vi "SwerveDriveLogic.vi"(8 "Z":dbl, 9 "Speeds":dbl[](array[numeric]), 10 "AngleSetpoints":dbl[](array[numeric]), 11 "AngleEncoders":dbl[](array[numeric])) -> (2 "AngleMotorsReversed":bool[](array[boolean]), 3 "AngleMotorOutputs":dbl[](array[numeric]))   [LabVIEW 2019]
uses:
  <vilib>/addons/control/pid/pid.llb/PID (DBL).vi
  <vilib>/addons/control/pid/NI_PID_pid.lvlib
panel:
  in  "PID gains":T1={"proportional gain (Kc)"=0.02, "integral time (Ti, min)"=0.0, "derivative time (Td, min)"=0.0} {"derivative time (Td, min)" format="%.15f"; "integral time (Ti, min)" format="%.3f"; "proportional gain (Kc)" format="%.3f"}
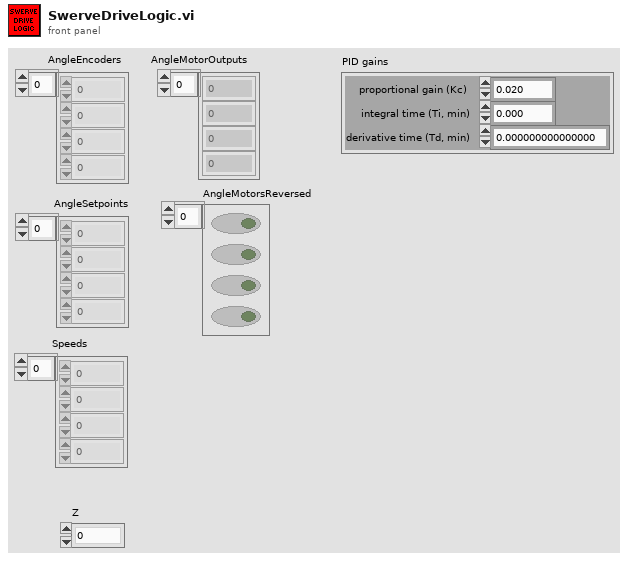
[diagram p1: front panel]
types:
  T1 = cluster{"proportional gain (Kc)":dbl, "integral time (Ti, min)":dbl, "derivative time (Td, min)":dbl}
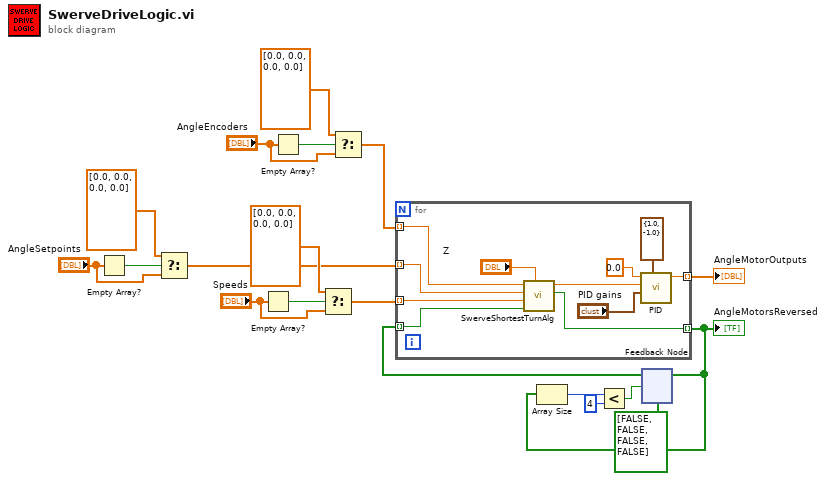
[diagram p0: block diagram]
diagram:
  n1 = Empty Array?(array="AngleSetpoints") -> (empty?=w16:bool)
  n2 = Select(t=dbl[] [0.0, 0.0, 0.0, 0.0] ("AngleSetpoints"), s=w16, f="AngleSetpoints") -> (s? t:f=w2:dbl[])
  n3 = Empty Array?(array="Speeds") -> (empty?=w14:bool)
  n4 = Empty Array?(array="AngleEncoders") -> (empty?=w19:bool)
  n5 = Select(t=dbl[] [0.0, 0.0, 0.0, 0.0] ("AngleSetpoints"), s=w14, f="Speeds") -> (s? t:f=w12:dbl[])
  n6 = Select(t=dbl[] [0.0, 0.0, 0.0, 0.0] ("AngleSetpoints"), s=w19, f="AngleEncoders") -> (s? t:f=w9:dbl[])
  n7 = feedback #1(bool[] [FALSE, FALSE, FALSE, FALSE]) -> (w5:bool[])
  n8 = for {
    tunnel: w5 -> [w25] mode=indexing
    tunnel: w2 -> [w27] mode=indexing
    tunnel: [w29] -> w1 mode=indexing
    tunnel: [w21] -> w4 mode=indexing
    tunnel: w9 -> [w24] mode=indexing
    tunnel: w12 -> [w23] mode=indexing
    n9 = call "SwerveShortestTurnAlg.vi"("Z"="Z", "SwerveMotorsFlipped?"=w25, "SwerveSpeed"=w23, "AngleSetpoint"=w27, "AngleEncoder"=w24) -> ("FlipSwerveMotors"=w21:bool, "PIDInput"=w22:dbl)  [unwired: 5 in]
    n10 = call-poly <vilib>:"PID.vi"("output range"=cluster{"output high":dbl, "output low":dbl} {"output high"=1.0, "output low"=-1.0}, "PID gains"="PID gains", "process variable"=w22, "setpoint"=0.0) -> ("output"=w29:dbl)  [unwired: 6 in, 1 out]
  }
  "AngleMotorsReversed" <- w4
  "AngleMotorOutputs" <- w1
  n11 = Array Size(array=w4) -> (size(s)=w6:i32)
  n12 = Less?(x=w6, y=4) -> (x < y?=w7:bool)
  n13 = feedback-in #1(w4, w7) -> ()
